vi "4145 Preview Plot.vi"(8 "error in (no error)":errorcluster, 11 "Spreadsheet data IN":T1) -> (0 "error out":errorcluster, 3 "Spreadsheet data OUT":T1)   [LabVIEW 2014]
uses:
  typedef/4145 Spreadsheet data.ctl
  <vilib>/Utility/miscctls.llb/LVRangeTypeDef.ctl
panel:
  in  "OK Button":bool
  out "graphics plot":cluster{dbl[], dbl[]}[](graph) caption="Plot Preview"
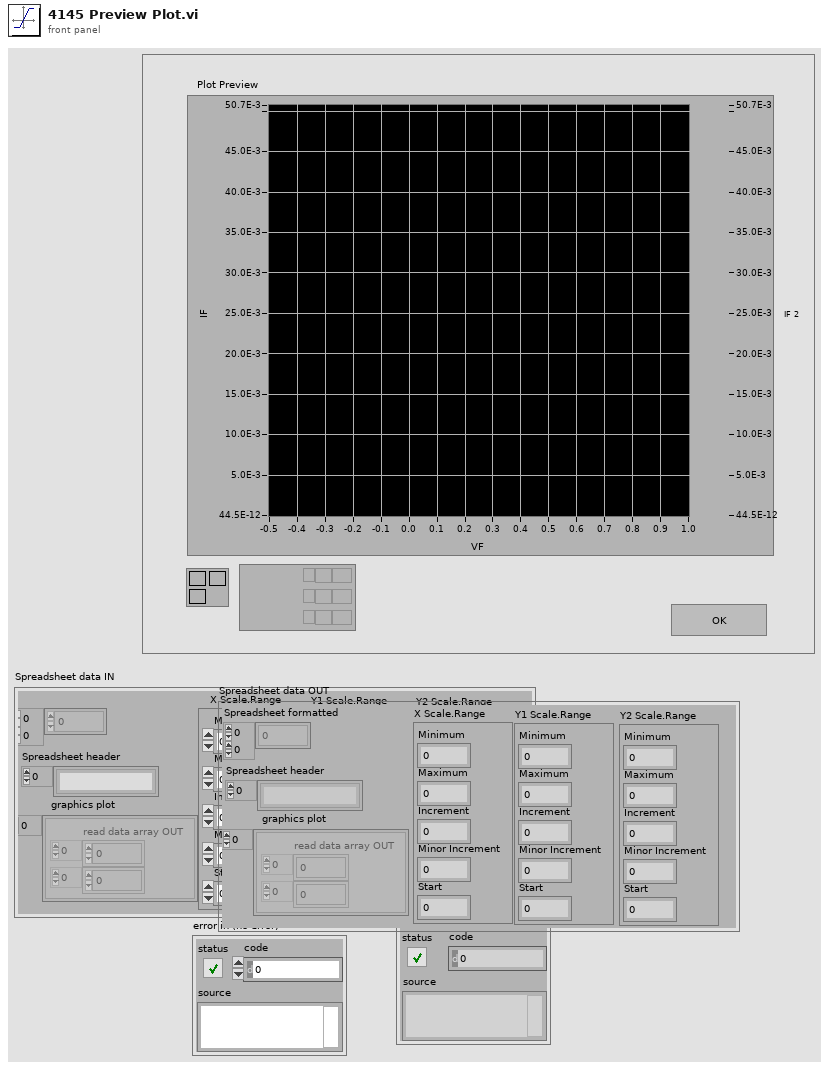
[diagram p1: front panel]
types:
  T1 = typedef "4145 Spreadsheet data.ctl" = cluster{"Spreadsheet formatted":dbl[][], "Spreadsheet header":string[], "graphics plot":cluster{"read data array OUT":dbl[], dbl[]}[], "X Scale.Range":T2, "Y1 Scale.Range ":T2, "Y2 Scale.Range":T2}
  T2 = typedef "LVRangeTypeDef.ctl" = cluster{"Minimum":dbl, "Maximum":dbl, "Increment":dbl, "Minor Increment":dbl, "Start":dbl}
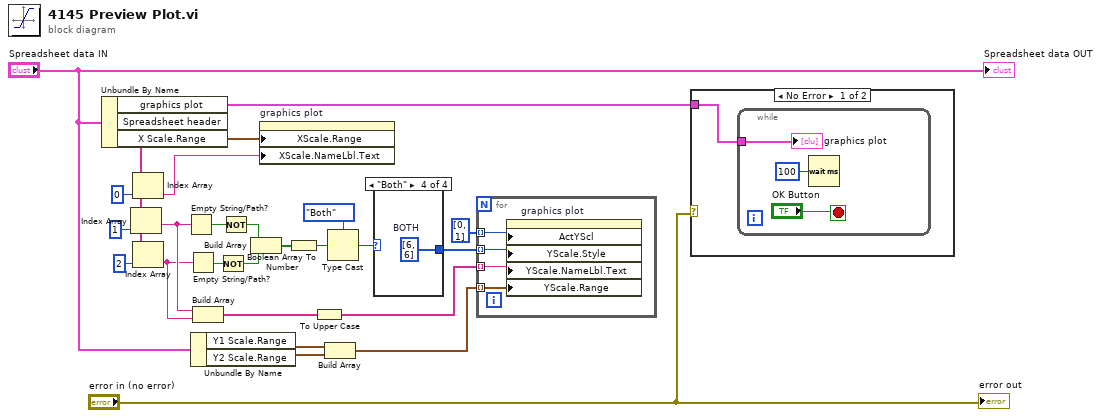
[diagram p0: block diagram]
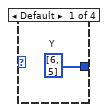
[diagram p2: hidden frame]
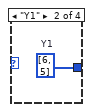
[diagram p3: hidden frame]
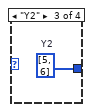
[diagram p4: hidden frame]
diagram:
  n1 = Unbundle By Name("Spreadsheet data IN") -> ("graphics plot"=w25:cluster{"read data array OUT":dbl[], dbl[]}[], "Spreadsheet header"=w10:string[], "X Scale.Range"=w5:T2)
  n2 = Index Array(array=w10, index=1) -> (element=w9:string)
  n3 = Index Array(array=w10, index=0) -> (element=w15:string)
  n4 = Index Array(array=w10, index=2) -> (element=w8:string)
  n5 = Empty String/Path?(string/path=w9) -> (empty?=w20:bool)
  n6 = Empty String/Path?(string/path=w8) -> (empty?=w19:bool)
  n7 = Unbundle By Name("Spreadsheet data IN") -> ("Y1 Scale.Range"=w3:T2, "Y2 Scale.Range"=w2:T2)
  n8 = Build Array(w9, w8) -> (w7:string[])
  n9 = Not(x=w19) -> (.not. x?=w16:bool)
  n10 = Not(x=w20) -> (.not. x?=w17:bool)
  n11 = Build Array(w17, w16) -> (w18:bool[])
  n12 = property on="graphics plot" class="XYGraph (strict)"("XScale.Range"=w5, "XScale.NameLbl.Text"=w15) -> ()  [unwired: 2 in, 2 out]
  n13 = Boolean Array To Number(Boolean array=w18) -> (number=w14:u32)
  n14 = To Upper Case(1:w7) -> (0:w6:string[])
  n15 = Build Array(w3, w2) -> (w1:T2[])
  n16 = Type Cast(type=enum16{"None", "Y1", "Y2", "Both"}."Both" ("Enum"), x=w14) -> (*(type *) &x=w13:enum16{"None", "Y1", "Y2", "Both"})
  n17 = case shown="\"Both\"" w13 {
    tunnel: [w27 w28 w29 w30] -> w21
    frame Default {
      w27 = i32[] [6, 5]  # Y
    }
    frame "Y1" {
      w28 = i32[] [6, 5]  # Y1
    }
    frame "Y2" {
      w29 = i32[] [5, 6]  # Y2
    }
    frame "Both" {
      w30 = i32[] [6, 6]  # BOTH
    }
  }
  n18 = for {
    tunnel: i32[] [0, 1] -> [w34] mode=indexing
    tunnel: w21 -> [w33] mode=indexing
    tunnel: w6 -> [w32] mode=indexing
    tunnel: w1 -> [w31] mode=indexing
    n19 = property on="graphics plot" class="XYGraph (strict)"("ActYScl"=w34, "YScale.Style"=w33, "YScale.NameLbl.Text"=w32, "YScale.Range"=w31) -> ()  [unwired: 2 in, 2 out]
  }
  n20 = case shown="No Error" "error in (no error)" {
    tunnel: w25 -> [w35 _]
    frame No Error {
      n21 = while {
        tunnel: w35 -> [w36]
        stop <- "OK Button" stop-if-true
        n22 = Wait (ms)(milliseconds to wait=u32 100) -> ()  [unwired: 1 out]
        "graphics plot" <- w36
      }
    }
    frame Error {
    }
  }
  "error out" <- "error in (no error)"
  "Spreadsheet data OUT" <- "Spreadsheet data IN"
